vi "test.vi"() -> ()   [LabVIEW 2021]
uses:
  Control 2.ctl
  <vilib>/myRIO/Common/Instrument Driver Framework/myRIO v1.0/PWM/vis/myRIO v1.0 Close PWM.vi
  <vilib>/myRIO/Common/Instrument Driver Framework/myRIO v1.0/PWM/vis/myRIO v1.0 Unreserve PWM.vi
  <vilib>/myRIO/Common/Instrument Driver Framework/myRIO v1.0/PWM/vis/myRIO v1.0 Build MUX Configuration PWM.vi
  <vilib>/myRIO/Common/Instrument Driver Framework/myRIO v1.0/Resource Manager/vis/myRIO v1.0 Unreserve Channel List.vi
  <vilib>/myRIO/Common/Instrument Driver Framework/myRIO v1.0/Resource Manager/vis/myRIO v1.0 Create Configuration List.vi
  <vilib>/myRIO/Common/Instrument Driver Framework/myRIO v1.0/Resource Manager/vis/myRIO v1.0 Unreserve Channel.vi
  <vilib>/myRIO/Common/Instrument Driver Framework/myRIO v1.0/Resource Manager/vis/myRIO v1.0 Build Mutex Name.vi
  <vilib>/Utility/error.llb/Error Cluster From Error Code.vi
  <vilib>/myRIO/Common/Instrument Driver Framework/myRIO v1.0/PWM/vis/myRIO v1.0 Write PWM.vi
  <vilib>/myRIO/Common/Instrument Driver Framework/myRIO v1.0/PWM/vis/myRIO v1.0 Shutdown PWM.vi
  <vilib>/myRIO/Common/Instrument Driver Framework/myRIO v1.0/Resource Manager/vis/myRIO v1.0 Configure IO.vi
  <vilib>/myRIO/Common/Instrument Driver Framework/Utilities/vis/Configuration Manager.vi
  <vilib>/myRIO/Common/Instrument Driver Framework/Utilities/vis/IO Manager.vi
  <vilib>/myRIO/Common/Instrument Driver Framework/myRIO v1.0/myRIO v1.0 Close.vi
  <vilib>/myRIO/Instrument Drivers/Onboard IO/PWM/PWM.lvlib
panel:
  out "Fan voltage":dbl
  out "Current State":T1
  in  "Duty Cycle":dbl(slide) scale=0.0..1.0
  in  "Setpoint":dbl(slide) scale=-40.0..50.0
  in  "Temp":dbl(slide) scale=-40.0..50.0
  in  "Frequency [Hz]":dbl(slide) scale=40.0..1000.0
  in  "stop":bool
  in  "error in (no error)":errorcluster
  out "error out":errorcluster
  # "(degC)"
  # "(degC)"
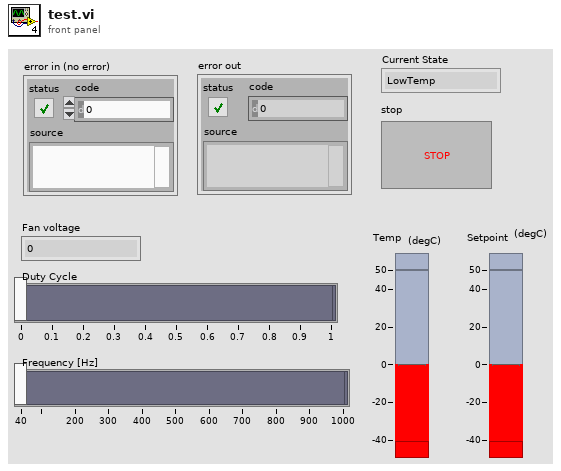
[diagram p1: front panel]
types:
  T1 = typedef "Control 2.ctl" = enum16{"LowTemp", "HighTemp", "Wait", "Shutdown"}
  T2 = typedef "PWM.lvlib/PWM Reference.ctl" = cluster{"myRIO Reference":T3, "PWM Channels Enum":T7, "PWM Configuration":T8}
  T3 = typedef "myRIO Generic Hardware Reference.ctl" = cluster{"myRIO Model":T4, "myRIO Hardware Reference":T5}
  T4 = typedef "Hardware Version Enum.ctl" = enum16{"Unknown", "myRIO-1900", "myRIO-1950", "roboRIO", "NI ELVIS RIO CM", "ELVIS III"}
  T5 = typedef "myRIO v1.0 Reference.ctl" = cluster{"Generic FPGA Reference":T6, "Allow multiple opens":bool}
  T6 = typedef "Generic FPGA Reference.ctl" = refnum<k20>
  T7 = typedef "PWM Channels Enum.ctl" = enum16{"Not Connected", "C/PWM0", "C/PWM1", "A/PWM0", "A/PWM1", "A/PWM2", "A/PWM3", "A/PWM4", "A/PWM5", "A/PWM6", "A/PWM7", "A/PWM8", "A/PWM9", "A/PWM10", "A/PWM11", "A/PWM12", "A/PWM13", "A/PWM14", "A/PWM15", "A/PWM16", "A/PWM17", "A/PWM18", "A/PWM19", "B/PWM0", "B/PWM1", "B/PWM2", "B/PWM3", "B/PWM4", "B/PWM5", "B/PWM6", "B/PWM7", "B/PWM8", "B/PWM9", "B/PWM10", "B/PWM11", "B/PWM12", "B/PWM13", "B/PWM14", "B/PWM15", "B/PWM16", "B/PWM17", "B/PWM18", "B/PWM19", "PWM/PWM0", "PWM/PWM1", "PWM/PWM2", "PWM/PWM3", "PWM/PWM4", "PWM/PWM5", "PWM/PWM6", "PWM/PWM7", "PWM/PWM8", "PWM/PWM9"}
  T8 = typedef "PWM.lvlib/PWM Configuration.ctl" = cluster{"Frequency":dbl, "Duty Cycle":dbl}
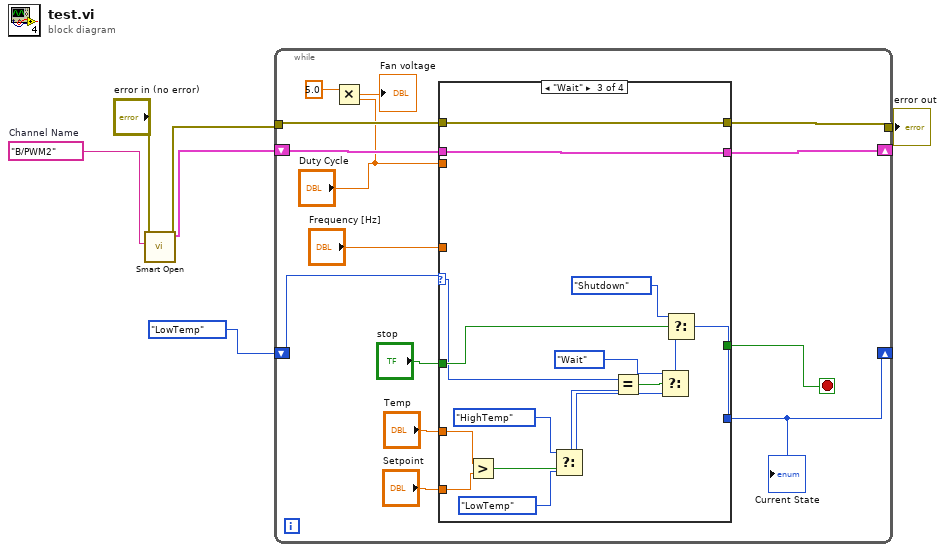
[diagram p0: block diagram]
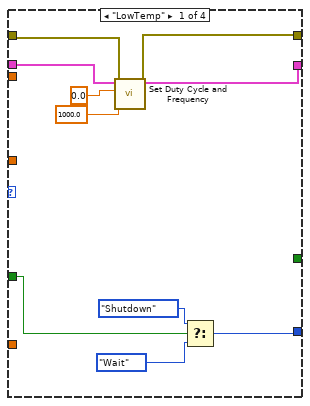
[diagram p2: hidden frame]
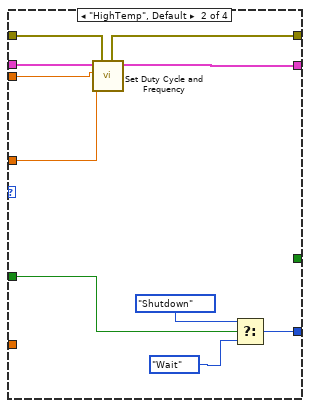
[diagram p3: hidden frame]
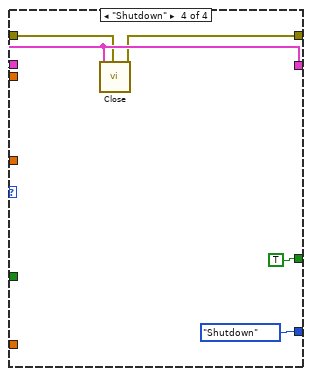
[diagram p4: hidden frame]
diagram:
  w4 = tag "B/PWM2"  # Channel Name
  n1 = call <vilib>:"Smart Open.vi"("error in (no error)"="error in (no error)", "Channel Name"=w4) -> ("error out"=w2:errorcluster, "PWM Ref Out"=w1:T2)  [unwired: 8 in]
  n2 = while {
    shift-right: [w19] -> _
    shift-left: Control_2."LowTemp" -> [w20]
    tunnel: [w13] -> w5
    tunnel: w2 -> [w16]
    shift-right: [w14] -> _
    shift-left: w1 -> [w15]
    stop <- w17 stop-if-true
    n3 = Multiply(x=5.0, y="Duty Cycle") -> (x*y=→"Fan voltage":dbl)
    n4 = case shown="\"Wait\"" w20 {
      selector: w20 -> [_ _ w45 _]
      tunnel: [w22 w33 w53 Control_2."Shutdown"] -> w19
      tunnel: "stop" -> [w23 w34 w54 _]
      tunnel: [_ _ _ TRUE] -> w17
      tunnel: w16 -> [w26 w38 w52 w57]
      tunnel: w15 -> [w30 w40 w51 w58]
      tunnel: "Duty Cycle" -> [_ w39 _ _]
      tunnel: [w29 w36 w51 w58] -> w14
      tunnel: [w25 w37 w52 w56] -> w13
      tunnel: "Temp" -> [_ _ w47 _]
      tunnel: "Setpoint" -> [_ _ w46 _]
      tunnel: "Frequency [Hz]" -> [_ w31 _ _]
      frame "LowTemp" {
        n5 = call <vilib>:"Set Duty Cycle and Frequency.vi"("error in (no error)"=w26, "Frequency [Hz]"=1000.0, "Duty Cycle"=0.0, "PWM Ref In"=w30) -> ("error out"=w25:errorcluster, "PWM Ref Out"=w29:T2)  [unwired: 5 in]
        n6 = Select(t=Control_2."Shutdown", s=w23, f=Control_2."Wait") -> (s? t:f=w22:T1)
      }
      frame "HighTemp", Default {
        n7 = call <vilib>:"Set Duty Cycle and Frequency.vi"("error in (no error)"=w38, "Frequency [Hz]"=w31, "Duty Cycle"=w39, "PWM Ref In"=w40) -> ("error out"=w37:errorcluster, "PWM Ref Out"=w36:T2)  [unwired: 5 in]
        n8 = Select(t=Control_2."Shutdown", s=w34, f=Control_2."Wait") -> (s? t:f=w33:T1)
      }
      frame "Wait" {
        n9 = Greater?(x=w47, y=w46) -> (0:w50:bool)
        n10 = Select(t=Control_2."HighTemp", s=w50, f=Control_2."LowTemp") -> (s? t:f=w42:T1)
        n11 = Equal?(x=w45, y=w42) -> (x = y?=w44:bool)
        n12 = Select(t=Control_2."Wait", s=w44, f=w42) -> (s? t:f=w41:T1)
        n13 = Select(t=Control_2."Shutdown", s=w54, f=w41) -> (s? t:f=w53:T1)
      }
      frame "Shutdown" {
        n14 = call <vilib>:"Close.vi"("error in (no error)"=w57, "PWM Ref In"=w58) -> ("error out"=w56:errorcluster)  [unwired: 9 in]
      }
    }
    "Current State" <- w19
  }
  "error out" <- w5
